vi "Dodana_energie.vi"() -> ()   [LabVIEW 2024]
uses:
  <vilib>/Analysis/baseanly.llb/Mean (DBL).vi
  <instrlib>/EFmeter/EFmeter.lvlib
  <vilib>/Analysis/NI_AALBase.lvlib
panel:
  in  "Cancel Button":bool
  out "Dodaná energie [Ws]":dbl
  in  "EFmeter VISA":refnum<visa-resource-name>
  in  "Adresa souboru":path
  in  "Prumerovani":bool
  in  "Vzorku na krokù":u32 max=100 step=1
  out "Zatezovaci charakteristika":cluster{"X":dbl[], "Y":dbl[]}[](graph)
  in  "Clear":bool
  in  "Ulozit data":bool caption="Uložit data"
  in  "Start":bool
  in  "stop":bool
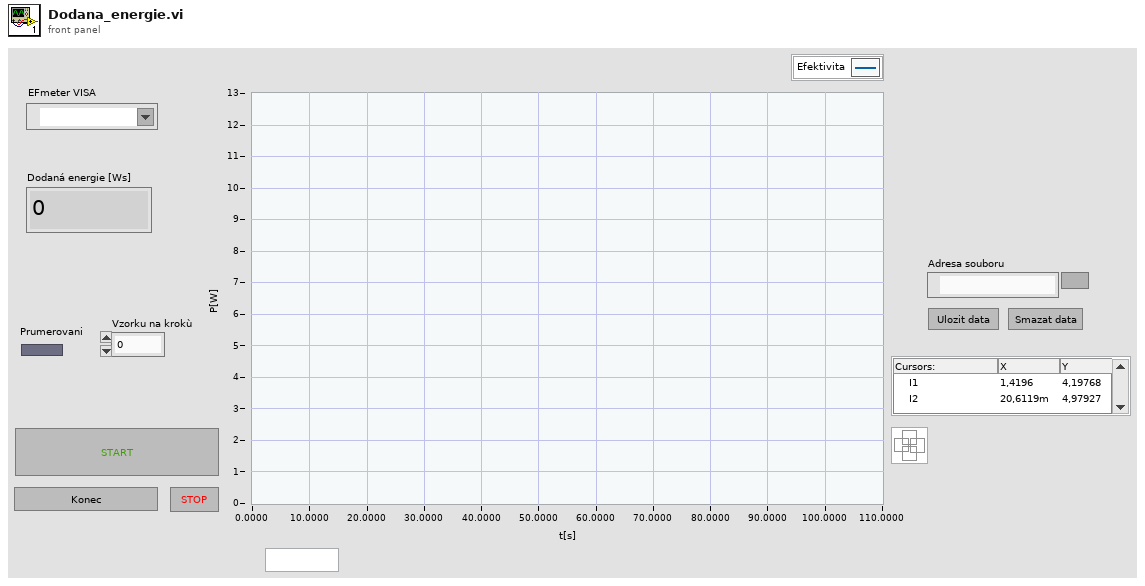
[diagram p1: front panel]
types:
  T1 = enum16{"open", "replace", "create", "open or create", "replace or create", "replace or create with confirmation"}
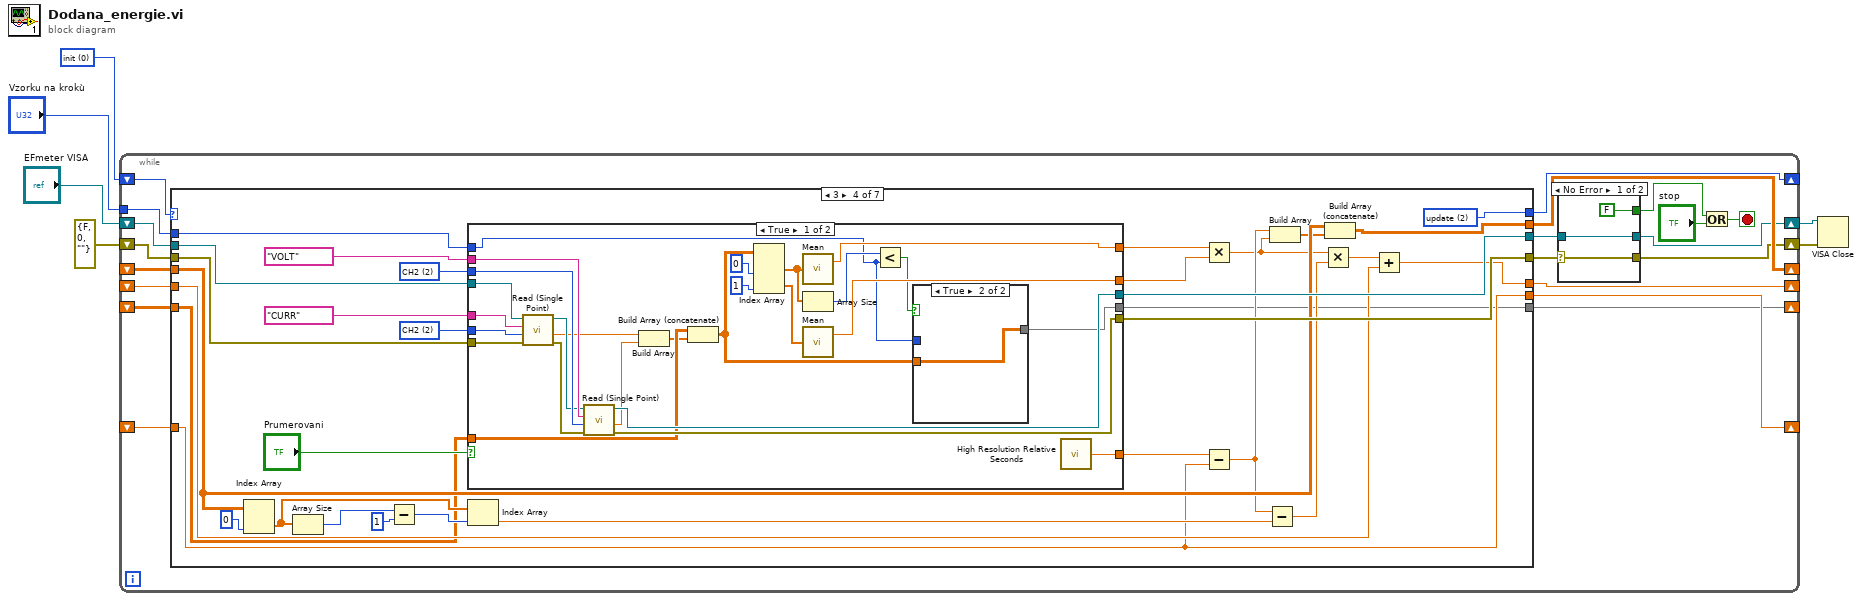
[diagram p0: block diagram]
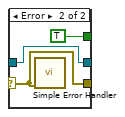
[diagram p2: hidden frame]
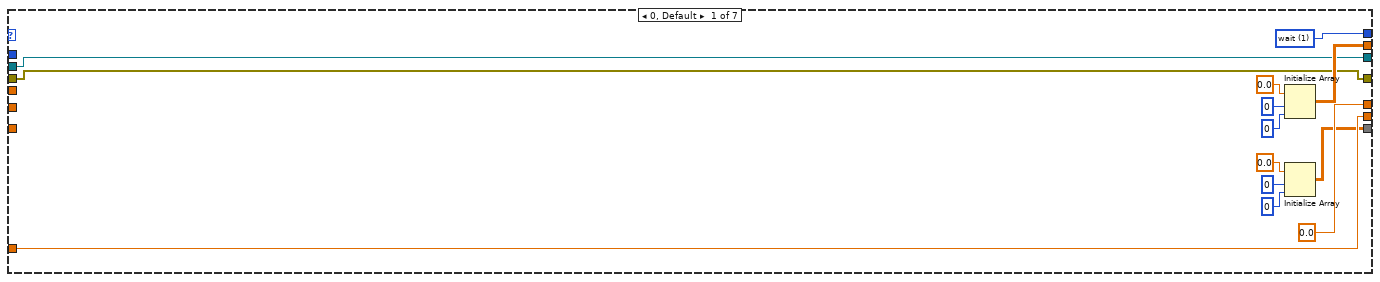
[diagram p3: hidden frame]
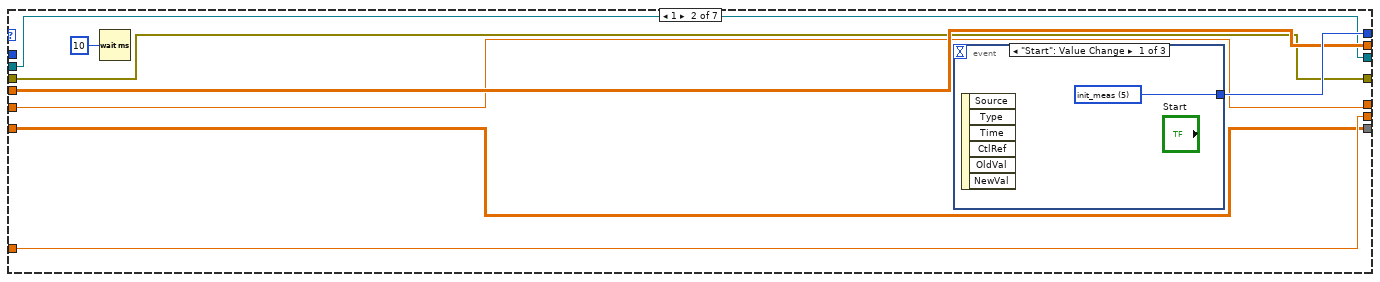
[diagram p4: hidden frame]
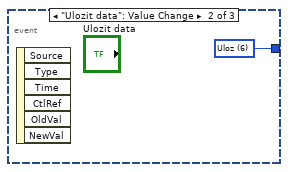
[diagram p5: hidden frame]
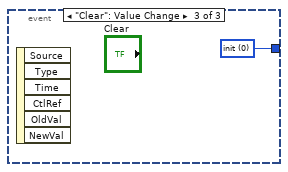
[diagram p6: hidden frame]
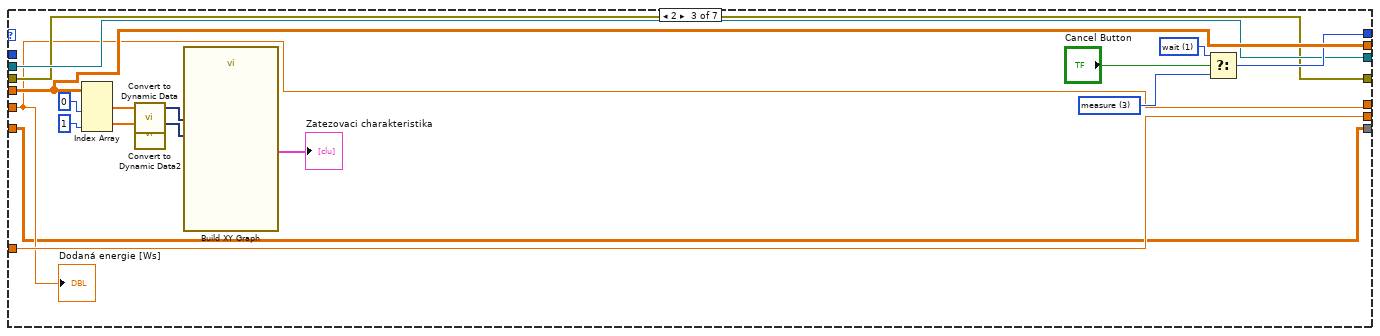
[diagram p7: hidden frame]
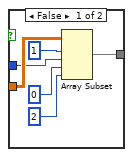
[diagram p8: hidden frame]
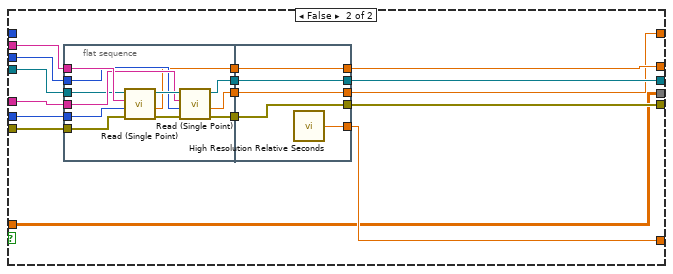
[diagram p9: hidden frame]
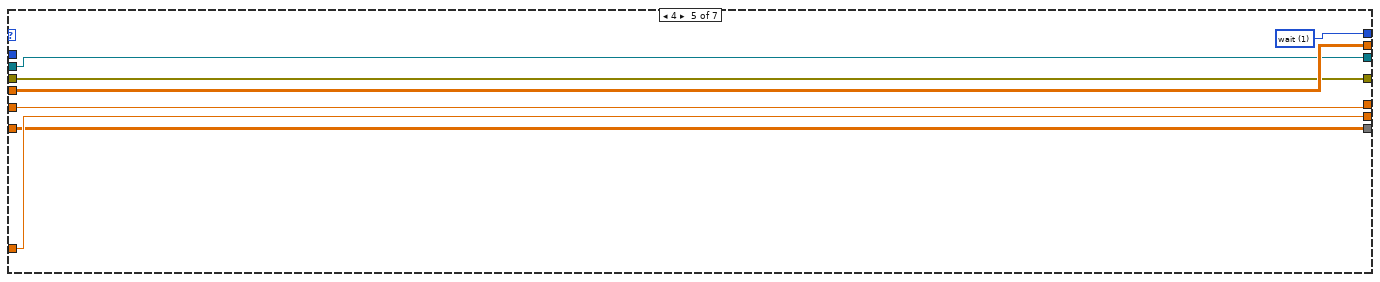
[diagram p10: hidden frame]
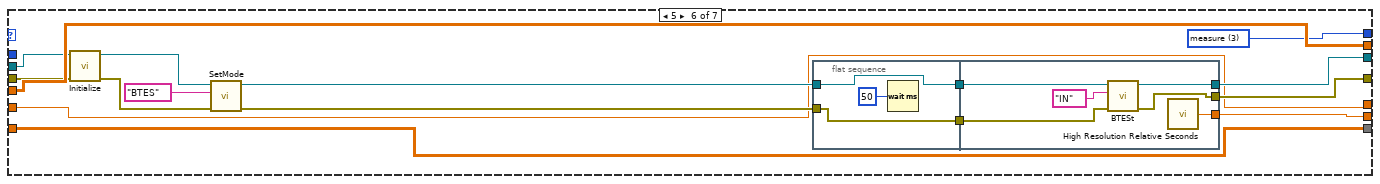
[diagram p11: hidden frame]
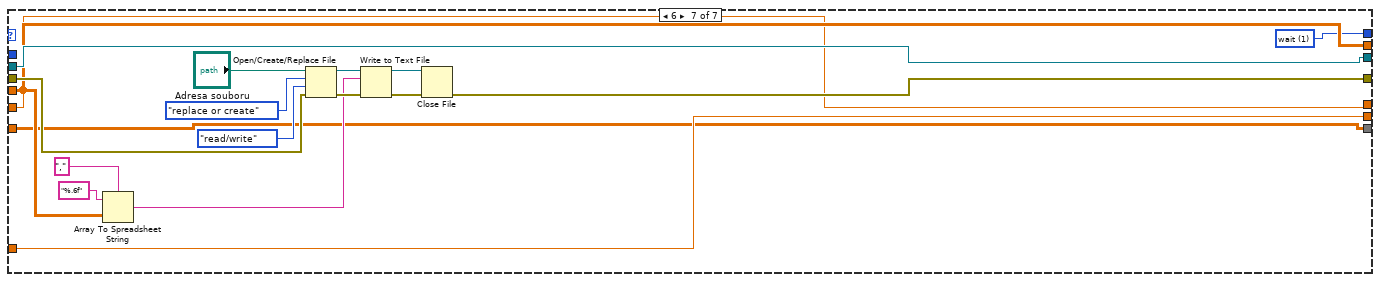
[diagram p12: hidden frame]
diagram:
  w6 = u16 0 items=["init", "wait", "update", "measure", "change_load", "init_meas", "Uloz", "clear"]
  n1 = while {
    shift-right: [w26] -> _
    shift-left: _ -> [w25]
    shift-right: [w21] -> _
    shift-left: w6 -> [w24]
    shift-right: [w18] -> w3
    shift-left: "EFmeter VISA" -> [w23]
    shift-right: [w17] -> w2
    shift-left: errorcluster {"status"=FALSE, "code"=0, "source"=""} ("error in (no error)") -> [w22]
    shift-right: [w13] -> _
    shift-left: _ -> [w12]
    shift-right: [w11] -> _
    shift-left: _ -> [w10]
    tunnel: "Vzorku na krokù" -> [w9]
    shift-right: [w8] -> _
    shift-left: _ -> [w7]
    stop <- w15 stop-if-true
    n2 = case shown="3" w24 {
      tunnel: [w43 w52 w68 w105 w178 w194 w216] -> w26
      tunnel: w25 -> [_ w52 w68 w93 w178 w194 w216]
      tunnel: [w42 w53 w67 w104 w173 w193 w214] -> w21
      tunnel: [w38 w50 w61 w100 w176 w183 w210] -> w20
      tunnel: [w41 w51 w62 w101 w177 w182 w221] -> w19
      tunnel: w23 -> [w41 w51 w62 w103 w177 w191 w221]
      tunnel: w22 -> [w38 w50 w61 w102 w176 w192 w217]
      tunnel: [w39 w48 w60 w77 w175 w181 w205] -> w13
      tunnel: w12 -> [w39 w48 w60 w77 w175 _ w205]
      tunnel: [0.0 w47 w59 w86 w174 w180 w206] -> w11
      tunnel: w10 -> [_ w47 w59 w87 w174 w180 w206]
      tunnel: w9 -> [_ _ _ w76 _ _ _]
      tunnel: [w33 w46 w57 w74 w172 w179 w204] -> w8
      tunnel: w7 -> [_ w46 w57 w75 w172 w179 w204]
      frame 0, Default {
        w42 = u16 1 items=["init", "wait", "update", "measure"]
        n3 = Initialize Array(0.0 ("element"), 0 ("dimension size"), 0 ("dimension size")) -> (w43:dbl[][])
        n4 = Initialize Array(0.0 ("element"), 0 ("dimension size"), 0 ("dimension size")) -> (w33:dbl[][])
      }
      frame 1 {
        n5 = Wait (ms)(milliseconds to wait=u32 10) -> ()  [unwired: 1 out]
        n6 = event shown="[0] \"Start\": Value Change" {
          selector: _ -> [_ _ _]
          dyn-events: _ -> [_ _ _]
          timeout: _ -> [_ _ _]
          tunnel: [w54 w55 w56] -> w53
          event "Start": Value Change {
            w54 = u16 5 items=["init", "wait", "update", "measure", "change_load", "init_meas"]
            n7 = event-data() -> ()  [unwired: 1 in, 6 out]
          }
          event "Ulozit data": Value Change {
            w55 = u16 6 items=["init", "wait", "update", "measure", "change_load", "init_meas", "Uloz"]
            n8 = event-data() -> ()  [unwired: 1 in, 6 out]
          }
          event "Clear": Value Change {
            w56 = u16 0 items=["init", "wait", "update", "measure", "change_load", "init_meas", "Uloz", "clear"]
            n9 = event-data() -> ()  [unwired: 1 in, 6 out]
          }
        }
      }
      frame 2 {
        w63 = u16 1 items=["init", "wait", "update", "measure", "change_load", "init_meas"]
        w69 = u16 3 items=["init", "wait", "update", "measure"]
        n10 = Index Array(array=w68, index (col) #1=0 ("index (row)"), index (col) #2=1 ("index (row)")) -> (element #1=w73:dbl[], element #2=w70:dbl[])  [unwired: 2 in]
        n11 = call "Convert to Dynamic Data"("Array"=w73) -> ("Dynamic Data Type"=w72:dynamicdata)  [unwired: 3 in]
        n12 = call "Convert to Dynamic Data2"("Array"=w70) -> ("Dynamic Data Type"=w71:dynamicdata)  [unwired: 3 in]
        n13 = call "Build XY Graph"("Y Input"=w71, "X Input"=w72) -> ("XY Graph"=→"Zatezovaci charakteristika":cluster{"X":dbl[], "Y":dbl[]}[])  [unwired: 8 in, 1 out]
        n14 = Select(t=w63, s="Cancel Button", f=w69) -> (s? t:f=w67:u16)
        "Dodaná energie [Ws]" <- w59
      }
      frame 3 {
        w95 = u16 2 items=["CH2"=2, "CH1"=1] ("Ring")
        w96 = u16 2 items=["CH2"=2, "CH1"=1] ("Ring")
        w104 = u16 2 items=["init", "wait", "update", "measure"]
        n15 = Index Array(array=w93, index (col)=0) -> (element=w92:dbl[])  [unwired: 1 in]
        n16 = Array Size(array=w92) -> (size(s)=w91:i32)
        n17 = Subtract(x=w91, y=1) -> (x-y=w90:i32)
        n18 = case shown="True" "Prumerovani" {
          tunnel: w103 -> [w121 w147]
          tunnel: w102 -> [w124 w148]
          tunnel: [w125 w154] -> w101
          tunnel: [w126 w153] -> w100
          tunnel: "VOLT" ("Combo Box") -> [w127 w152]
          tunnel: "CURR" ("Combo Box") -> [w122 w150]
          tunnel: w96 -> [w128 w149]
          tunnel: w95 -> [w123 w151]
          tunnel: [w129 w140] -> w82
          tunnel: [w130 w146] -> w80
          tunnel: [w131 w145] -> w79
          tunnel: w76 -> [w106 _]
          tunnel: w75 -> [w112 w139]
          tunnel: [w107 w139] -> w74
          frame True {
            n19 = call <instrlib>:"Read (Single Point).vi"("error in (no error)"=w124, "Ring"=w123, "Combo Box"=w122, "VISA resource name"=w121) -> ("error out"=w120:errorcluster, "Measurement"=w118:dbl, "VISA resource name out"=w119:refnum<visa-resource-name>)  [unwired: 5 in]
            n20 = call <instrlib>:"Read (Single Point).vi"("error in (no error)"=w120, "Ring"=w128, "Combo Box"=w127, "VISA resource name"=w119) -> ("error out"=w126:errorcluster, "Measurement"=w117:dbl, "VISA resource name out"=w125:refnum<visa-resource-name>)  [unwired: 5 in]
            n21 = Build Array(w118, w117) -> (w111:dbl[])
            n22 = Build Array (concatenate)(w112, w111) -> (w110:dbl[][])
            n23 = Index Array(array=w110, index (col) #1=0 ("index (col)"), index (col) #2=1 ("index (col)")) -> (element #1=w108:dbl[], element #2=w109:dbl[])  [unwired: 2 in]
            n24 = call-poly <vilib>:"Mean.vi"("X"=w108) -> ("mean"=w131:dbl)  [unwired: 1 out]
            n25 = Array Size(array=w108) -> (size(s)=w114:i32)
            n26 = call-poly <vilib>:"Mean.vi"("X"=w109) -> ("mean"=w130:dbl)  [unwired: 1 out]
            n27 = Less?(x=w114, y=w106) -> (x < y?=w113:bool)
            n28 = case shown="True" w113 {
              tunnel: w110 -> [w134 w138]
              tunnel: [w133 w138] -> w107
              tunnel: w106 -> [w132 _]
              frame False {
                n29 = Array Subset(array=w134, index (row)=1 ("index"), length (row)=w132, index (col)=0 ("index"), length (col)=2 ("length")) -> (w133:dbl[][])
              }
              frame True {
              }
            }
            n30 = call <vilib>:"High Resolution Relative Seconds.vi"() -> ("relative seconds"=w129:dbl)
          }
          frame False {
            n31 = flat-sequence {
              tunnel: w152 -> [w162]
              tunnel: w151 -> [w161]
              tunnel: w150 -> [w160]
              tunnel: w149 -> [w159]
              tunnel: w148 -> [w158]
              tunnel: w147 -> [w157]
              tunnel: [w164] -> w144
              tunnel: [w163] -> w143
              tunnel: [w156] -> w142
              tunnel: [w155] -> w141
              tunnel: [w168] -> w145
              tunnel: [w169] -> w146
              tunnel: [w170] -> w153
              tunnel: [w171] -> w154
              tunnel: w144 -> [w171]
              tunnel: w143 -> [w170]
              tunnel: w142 -> [w169]
              tunnel: w141 -> [w168]
              tunnel: [w167] -> w140
              frame #0 {
                n32 = call <instrlib>:"Read (Single Point).vi"("error in (no error)"=w158, "Ring"=w161, "Combo Box"=w162, "VISA resource name"=w157) -> ("error out"=w165:errorcluster, "Measurement"=w156:dbl, "VISA resource name out"=w166:refnum<visa-resource-name>)  [unwired: 5 in]
                n33 = call <instrlib>:"Read (Single Point).vi"("error in (no error)"=w165, "Ring"=w159, "Combo Box"=w160, "VISA resource name"=w166) -> ("error out"=w163:errorcluster, "Measurement"=w155:dbl, "VISA resource name out"=w164:refnum<visa-resource-name>)  [unwired: 5 in]
              }
              frame #1 {
                n34 = call <vilib>:"High Resolution Relative Seconds.vi"() -> ("relative seconds"=w167:dbl)
              }
            }
          }
        }
        n35 = Index Array(array=w92, index=w90) -> (element=w84:dbl)
        n36 = Multiply(x=w79, y=w80) -> (x*y=w78:dbl)
        n37 = Subtract(x=w82, y=w77) -> (x-y=w81:dbl)
        n38 = Subtract(x=w81, y=w84) -> (x-y=w83:dbl)
        n39 = Build Array(w81, w78) -> (w88:dbl[])
        n40 = Multiply(x=w78, y=w83) -> (x*y=w85:dbl)
        n41 = Build Array (concatenate)(w93, w88) -> (w105:dbl[][])
        n42 = Add(x=w85, y=w87) -> (x+y=w86:dbl)
      }
      frame 4 {
        w173 = u16 1 items=["init", "wait", "update", "measure", "change_load", "init_meas", "Uloz", "clear"]
      }
      frame 5 {
        w193 = u16 3 items=["init", "wait", "update", "measure", "change_load", "init_meas"]
        n43 = call <instrlib>:"Initialize.vi"("error in (no error)"=w192, "VISA resource name"=w191) -> ("error out"=w188:errorcluster, "VISA resource name out"=w189:refnum<visa-resource-name>)  [unwired: 8 in]
        n44 = call <instrlib>:"SetMode.vi"("error in (no error)"=w188, "Combo Box"="BTES", "VISA resource name"=w189) -> ("error out"=w187:errorcluster, "VISA resource name out"=w186:refnum<visa-resource-name>)  [unwired: 7 in]
        n45 = flat-sequence {
          tunnel: w186 -> [w196]
          tunnel: w187 -> [w195]
          tunnel: [w196] -> w185
          tunnel: [w195] -> w184
          tunnel: w185 -> [w202]
          tunnel: w184 -> [w203]
          tunnel: [w201] -> w183
          tunnel: [w200] -> w182
          tunnel: [w198] -> w181
          frame #0 {
            n46 = Wait (ms)(milliseconds to wait=u32 50) -> ()  [unwired: 1 out]
          }
          frame #1 {
            n47 = call <instrlib>:"BTESt.vi"("error in (no error)"=w203, "Combo Box"="IN", "VISA resource name"=w202) -> ("error out"=w201:errorcluster, "VISA resource name out"=w200:refnum<visa-resource-name>)  [unwired: 7 in]
            n48 = call <vilib>:"High Resolution Relative Seconds.vi"() -> ("relative seconds"=w198:dbl)
          }
        }
      }
      frame 6 {
        w214 = u16 1 items=["init", "wait", "update", "measure", "change_load", "init_meas"]
        n49 = Array To Spreadsheet String(delimiter (Tab)=",", array=w216, 3:"%.6f" ("format string")) -> (spreadsheet string=w207:string)
        n50 = Open/Create/Replace File(file path (use dialog)="Adresa souboru", error in=w217, operation (0:open)=T1."replace or create", access (0:read/write)=enum16{"read/write", "read-only", "write-only"}."read/write") -> (refnum out=w209:refnum<file>, error out=w212:errorcluster)  [unwired: 2 in, 1 out]
        n51 = Write to Text File(file (use dialog)=w209, text=w207, error in=w212) -> (refnum out=w208:refnum<file>, error out=w211:errorcluster)  [unwired: 1 in, 1 out]
        n52 = Close File(refnum=w208, error in=w211) -> (error out=w210:errorcluster)  [unwired: 1 out]
      }
    }
    n53 = case shown="No Error" w20 {
      selector: w20 -> [w28 w30]
      tunnel: w19 -> [w29 w32]
      tunnel: [w29 w32] -> w18
      tunnel: [w28 w30] -> w17
      tunnel: [FALSE TRUE] -> w14
      frame No Error {
      }
      frame Error {
        n54 = call <vilib>:"Simple Error Handler.vi"("error in (no error)"=w30) -> ()  [unwired: 4 in, 5 out]
      }
    }
    n55 = Or(x=w14, y="stop") -> (x .or. y?=w15:bool)
  }
  n56 = VISA Close(VISA resource name=w3, error in (no error)=w2) -> ()  [unwired: 1 out]
